vi "Write CSV File.vi"   [LabVIEW 2012, in "Robust CSV.lvlib"]
uses:
  <userlib>/Robust CSV/Robust CSV.lvlib
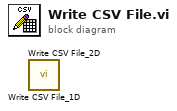
[diagram p0: block diagram]
diagram:
  n1 = call <userlib>:"Write CSV File_1D.vi"() -> ()  [unwired: 10 in, 2 out]
  n2 = call <userlib>:"Write CSV File_2D.vi"() -> ()  [unwired: 10 in, 2 out]
